vi "Channel Validation.vi"(8 "error in (no error)":errorcluster, 10 "Channel in":T1, 11 "EPU452 in":refnum<class "EPU452.lvclass">) -> (0 "error out":errorcluster, 1 "Channel":string, 2 "Is Channel Valid?":bool, 3 "EPU452 out":refnum<class "EPU452.lvclass">)   [LabVIEW 2018, in "EPU452.lvclass"]
uses:
  EPU452.lvclass
  Controls/Channels.ctl
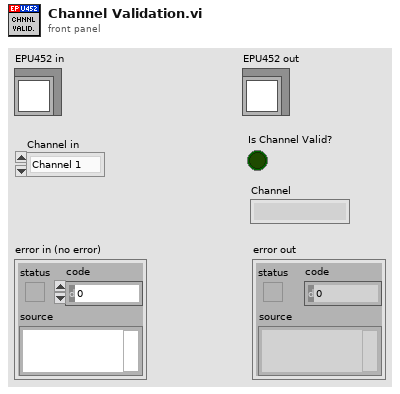
[diagram p1: front panel]
types:
  T1 = typedef "EPU452.lvclass/Channels.ctl" = enum16{"Channel 1", "Channel 2", "Channel 3", "Channel 4"}
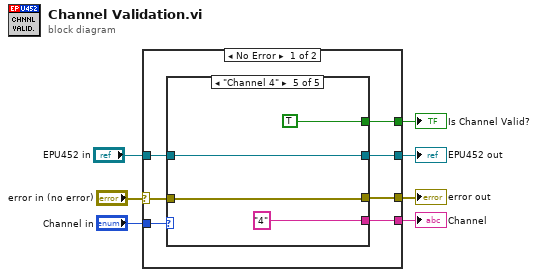
[diagram p0: block diagram]
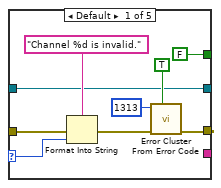
[diagram p2: hidden frame]
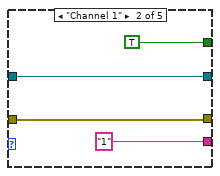
[diagram p3: hidden frame]
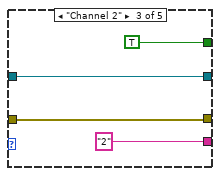
[diagram p4: hidden frame]
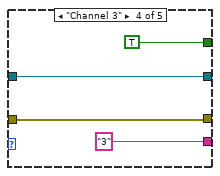
[diagram p5: hidden frame]
diagram:
  n1 = case shown="No Error" "error in (no error)" {
    selector: "error in (no error)" -> [w12 w41]
    tunnel: [w11 w41] -> w6
    tunnel: [w10 w40] -> w4
    tunnel: "EPU452 in" -> [w13 w40]
    tunnel: "Channel in" -> [w14 _]
    tunnel: [w9 _] -> w2
    tunnel: [w8 _] -> w1
    frame No Error {
      n2 = case shown="\"Channel 4\"" w14 {
        selector: w14 -> [w16 _ _ _ _]
        tunnel: w13 -> [w17 w27 w31 w35 w39]
        tunnel: w12 -> [w19 w26 w30 w34 w38]
        tunnel: [w18 w26 w30 w34 w38] -> w11
        tunnel: [w17 w27 w31 w35 w39] -> w10
        tunnel: [FALSE ("show call chain? (False)") TRUE ("show call chain? (False)") TRUE ("show call chain? (False)") TRUE ("show call chain? (False)") TRUE ("show call chain? (False)")] -> w9
        tunnel: [_ "1" "2" "3" "4"] -> w8
        frame Default {
          n3 = Format Into String(format string="Channel %d is invalid.", error in=w19, w16) -> (error out=w22:errorcluster)  [unwired: 1 in, 1 out]
          n4 = call <vilib>:"Error Cluster From Error Code.vi"("show call chain? (False)"=TRUE, "error in (no error)"=w22, "error code (0)"=1313) -> ("error out"=w18:errorcluster)  [unwired: 6 in]
        }
        frame "Channel 1" {
        }
        frame "Channel 2" {
        }
        frame "Channel 3" {
        }
        frame "Channel 4" {
        }
      }
    }
    frame Error {
    }
  }
  "error out" <- w6
  "EPU452 out" <- w4
  "Is Channel Valid?" <- w2
  "Channel" <- w1
